vi "Publish Test Value.vi"(8 "error in (no error)":errorcluster, 11 "RootModelPublishesDoubleFloat In":refnum<class "RootModelPublishesDoubleFloat.lvclass">) -> (0 "error out":errorcluster, 3 "RootModelPublishesDoubleFloat Out":refnum<class "RootModelPublishesDoubleFloat.lvclass">)   [LabVIEW 2020, in "RootModelPublishesDoubleFloat.lvlib" / "RootModelPublishesDoubleFloat.lvclass"]
uses:
  RootModelPublishesDoubleFloat.lvclass
  RootModelPublishesDoubleFloat.lvclass/RootModelPublishesDoubleFloat.ctl
  Source/IModel/IModel/IModel.lvclass
  C:/Git/mva-core/Source/RootModel/RootModel/RootModel.lvclass
  C:/Git/mva-core/Source/IModel/IModel/IModel.lvclass
  C:/Git/mva-core/Source/IObserver/IObserver/IObserver.lvclass
  C:/Program Files (x86)/National Instruments/LabVIEW 2020/vi.lib/ActorFramework/Actor/Actor.lvclass
  C:/Git/mva-core/Test/Doubles/RootModelPublishesDoubleFloat/RootModelPublishesDoubleFloat.lvclass
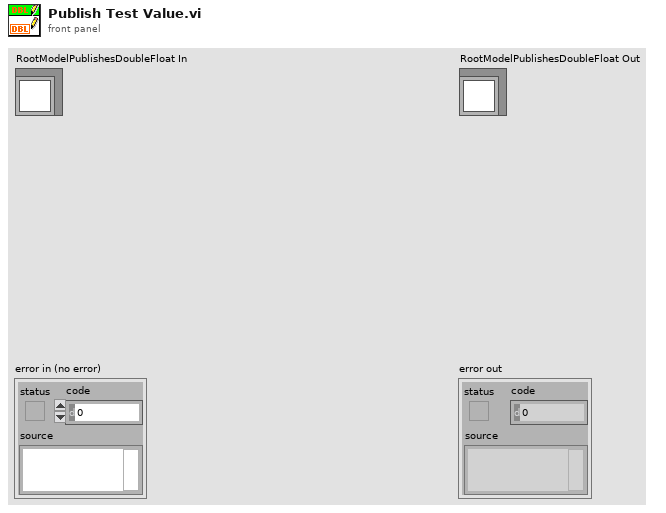
[diagram p1: front panel]
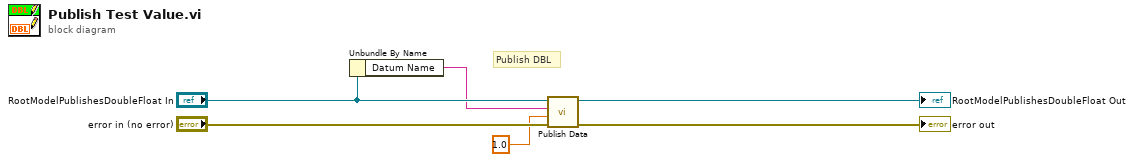
[diagram p0: block diagram]
diagram:
  # "Publish DBL"
  n1 = Unbundle By Name("RootModelPublishesDoubleFloat In") -> ("Datum Name"=w1:string)
  n2 = call "Publish Data.vi"("error in (no error)"="error in (no error)", "Data to Publish"=1.0, "Datum Name"=w1, "IModel in"="RootModelPublishesDoubleFloat In") -> ("error out"=→"error out":errorcluster, "IModel out"=→"RootModelPublishesDoubleFloat Out":refnum<class "RootModelPublishesDoubleFloat.lvclass">)  [unwired: 6 in]
